vi "get_physical_channel.vi"(8 "error in (no error)":errorcluster, 11 "DAQmxAnalogOut in":refnum<class "AnalogOutDL101207DAQmx.lvclass">) -> (0 "error out":errorcluster, 2 "DAQmx Physical Channel":tag, 3 "DAQmxAnalogOut out":refnum<class "AnalogOutDL101207DAQmx.lvclass">)   [LabVIEW 2010, in "AnalogOutDL101207DAQmx.lvclass"]
uses:
  AnalogOutDL101207DAQmx.lvclass
  AnalogOutDL101207DAQmx.lvclass/AnalogOutDL101207DAQmx.ctl
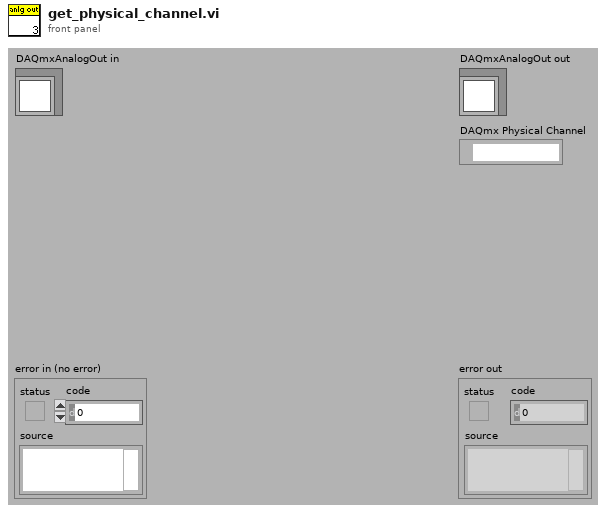
[diagram p1: front panel]
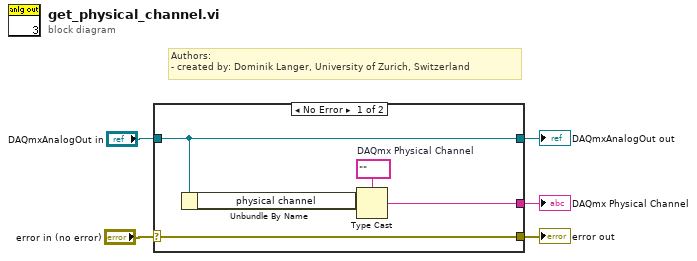
[diagram p0: block diagram]
diagram:
  # "Authors: \n- created by: Dominik Langer, University of Zurich, Switzerland"
  n1 = case shown="No Error" "error in (no error)" {
    selector: "error in (no error)" -> [w10 w12]
    tunnel: [w10 w12] -> w4
    tunnel: [w9 w11] -> w2
    tunnel: "DAQmxAnalogOut in" -> [w9 w11]
    tunnel: [w6 _] -> w1
    frame No Error {
      w7 = tag ""  # DAQmx Physical Channel
      n2 = Unbundle By Name(w9) -> ("physical channel"=w8:string)
      n3 = Type Cast(type=w7, x=w8) -> (*(type *) &x=w6:tag)
    }
    frame Error {
    }
  }
  "error out" <- w4
  "DAQmxAnalogOut out" <- w2
  "DAQmx Physical Channel" <- w1
